vi "Target_4651.vi"() -> ()   [LabVIEW 2018]
uses:
  <vilib>/Platform/TimedLoop/XDataNode/timing_clust.ctl
  <vilib>/Platform/TimedLoop/XDataNode/nitl_modes.ctl
  <vilib>/Platform/TimedLoop/XDataNode/wakeup.ctl
  <vilib>/rvi/eio/common/nirviEmuTemplateMethod_errors.vi
  <vilib>/rvi/Emulation/niFpgaGetClockAttributes.vi
  <vilib>/rvi/Emulation/niFpgaSctlEmulationGetInTimedLoop.vi
  <vilib>/rvi/Emulation/niFpgaEmulationReportErrorSimple.vi
  <vilib>/rvi/Emulation/niFpgaProcessEmulError.vi
  <vilib>/rvi/Emulation/niFpgaCriticalErrorInLSC.vi
  <vilib>/rvi/Memory/Memory_Emulation/niFpgaMemoryFastEmulationDramWriteAndRequestData.vi
  <vilib>/rvi/Memory/Memory_Emulation/niFpgaMemoryEmulationDramWriteAndRequestData.vi
  <vilib>/rvi/DataTransferAndStorage/Container/Common/niFpgaContainerGetUniqueNameForEmu.vi
  <vilib>/rvi/Memory/Memory_Emulation/niFpgaMemoryEmulationDramWriteAndRequestDataApplyByteEnables.vi
  <vilib>/rvi/Memory/Memory_Emulation/nirvimemoryFastEmulation.vi
  <vilib>/rvi/Memory/Memory_Emulation/nirvimemoryEmulation.vi
  <vilib>/rvi/Emulation/niFpgaEmulationIsFPGAContextNoSignature.vi
  <vilib>/rvi/errors/nirviReportUnexpectedCaseInternalError (U32).vi
  <vilib>/rvi/interface/RandomDataEmulation/niFpgaRandomDataHandleErrors.vi
  <vilib>/eio/EIONode/EIONode.xnode
  <vilib>/Platform/TimedLoop/XDataNode/XDataNode.xnode
  <vilib>/rvi/DataTransferAndStorage/Container/XNode/niFpgaContainer.xnode
  <vilib>/rvi/interface/RandomDataEmulation/nirviRandomDataFpgaReadWriteTemplate.vi
  <vilib>/rvi/Memory/Memory_Emulation/niFpgaMemoryEmulationDramRetrieveData.vi
  <vilib>/Platform/TimedLoop/XDataNode/XDNodeRunTimeDep.lvlib
  <instrlib>/_niInstr/Basic Elements/v1/FPGA/niInstr Basic Elements v1 FPGA.lvlib
panel:
  in  "EOL":u64=281406257234029
  in  "SOL":u64=281406257234133
  in  "EOF":u64=281406257234105
  in  "SOF":u64=281406257233921
  in  "FR":u8=19
  in  "Кол-во":u16=370
  in  "Адрес":u16
  out "Записали адресов":u32
  in  "3924360":u32=3924360
  in  "48":u8=48
  in  "48":bool[](array[boolean])=[FALSE, FALSE, FALSE, FALSE, FALSE, FALSE, FALSE, FALSE, FALSE, FALSE, FALSE, FALSE, FALSE, FALSE, FALSE, FALSE, FALSE, FALSE, FALSE, FALSE, FALSE, FALSE, FALSE, FALSE, FALSE, FALSE, FALSE, FALSE, FALSE, FALSE, FALSE, FALSE, FALSE, FALSE, FALSE, FALSE, FALSE, FALSE, FALSE, FALSE, FALSE, FALSE, FALSE, FALSE, FALSE, FALSE, FALSE, FALSE]
  in  "Кадр в память":bool
  in  "Кадр на ПК":bool
  in  "Нач_адр":u32
  in  "Кон_адр":u32=32703
  out "Записали FIFO":bool
  in  "Автомат":bool
  in  "SYS_RST_N":bool
  in  "Стоп":bool
  out "SPI_OFF":bool
  in  "12":u8=12
  in  "W(T)/R(F)":bool
  in  "19":u8=19
  in  "SPI":bool
  in  "Upd_WR":bool
  in  "369":u16=369
  in  "Upd_RD":bool
  in  "372":u16=372
  in  "370":u16=370
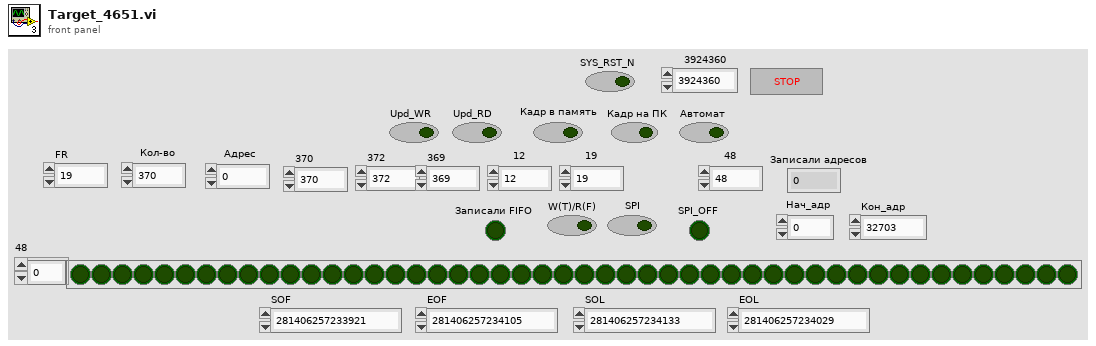
[diagram p1: front panel]
types:
  T1 = typedef "XDNodeRunTimeDep.lvlib/timing_clust.ctl" = cluster{"Expected End [f-1]":u64, "Actual End [f-1]":u64, "Finished Late? [f-1]":bool, "Expected End [i-1]":u64, "Actual End [i-1]":u64, "Finished Late? [i-1]":bool, "Expected Start [i]":u64, "Actual Start [i]":u64, "Expected Start [f]":u64, "Actual Start [f]":u64, "Source Name":string, "Structure Name":string, "Period":i64, "Deadline":i64, "Offset":i64, "Start":i64, "Priority":i32, "Timeout":i32, "Mode":T2, "Wakeup Reason":T3, "Error":errorcluster, "Source Type":string, "Secondary Source Type":string, "Global End Time":u64, "Global Start Time":u64, "Frame Duration":u64, "Iteration Duration":u64, "Assigned CPU":i32, "I/O Scan Engine Mode":u32}
  T2 = typedef "XDNodeRunTimeDep.lvlib/nitl_modes.ctl" = enum32{"No Change", "Process missed periods, maintain original phase", "Discard missed periods, maintain original phase", "Process missed periods, ignore original phase", "Discard missed periods, ignore original phase"}
  T3 = typedef "XDNodeRunTimeDep.lvlib/wakeup.ctl" = enum32{"Normal", "Aborted", "Asynchronous wakeup", "Timing source error", "Timed loop error", "Timeout"}
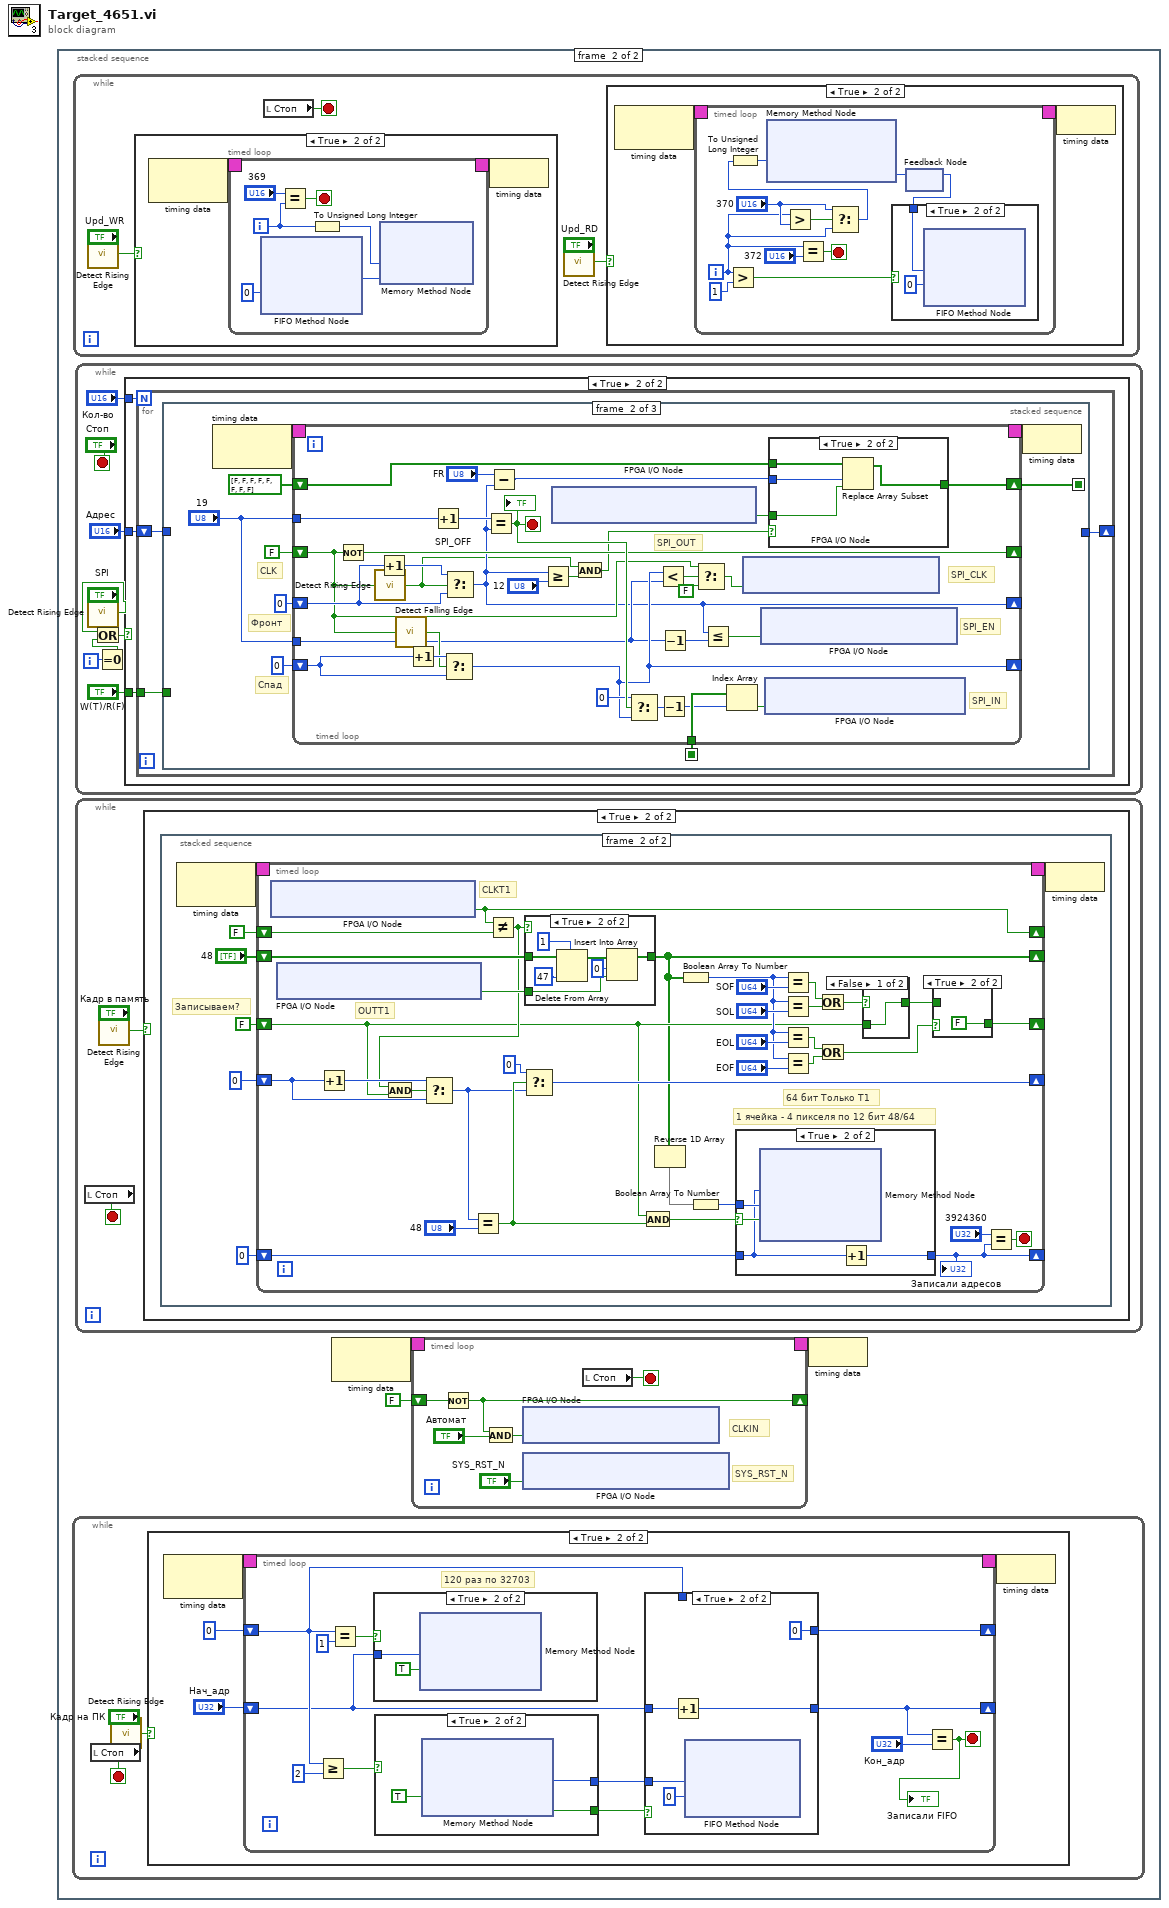
[diagram p0: block diagram]
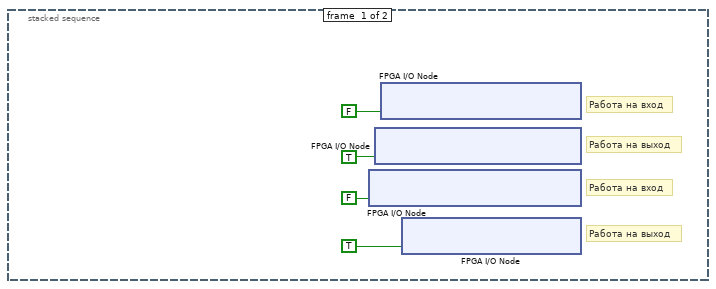
[diagram p2: hidden frame]
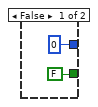
[diagram p4: hidden frame]
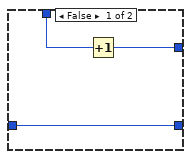
[diagram p6: hidden frame]
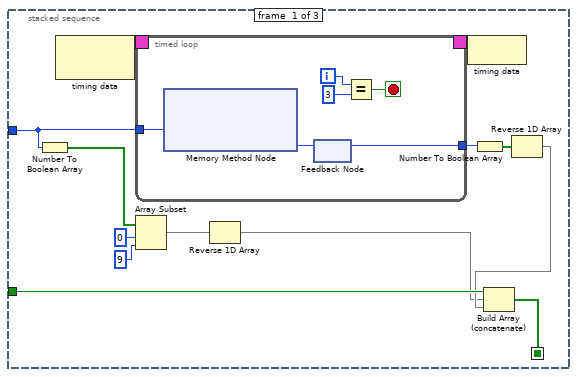
[diagram p11: hidden frame]
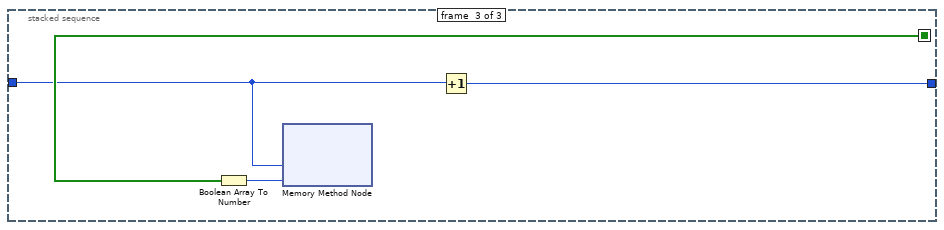
[diagram p13: hidden frame]
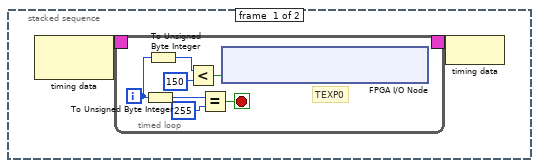
[diagram p15: hidden frame]
diagram:
  n1 = stacked-sequence {
    frame #0 {
      # "Работа на выход"
      # "Работа на вход"
      # "Работа на выход"
      # "Работа на вход"
      n2 = xnode "FPGA I/O Node"("IO Module\\DDCA_DIO16-23_WE"=FALSE ("IO Module\\DDCA_DIO16-23_WE")) -> ()  [unwired: 1 in, 1 out]
      n3 = xnode "FPGA I/O Node"("IO Module\\DDCA_DIO8-15_WE"=TRUE ("IO Module\\DDCA_DIO8-15_WE")) -> ()  [unwired: 1 in, 1 out]
      n4 = xnode "FPGA I/O Node"("IO Module\\DDCA_DIO0-7_WE"=FALSE ("IO Module\\DDCA_DIO0-7_WE")) -> ()  [unwired: 1 in, 1 out]
      n5 = xnode "FPGA I/O Node"("IO Module\\DDCA_PFI_WE"=TRUE ("IO Module\\DDCA_DIO16-23_WE")) -> ()  [unwired: 1 in, 1 out]
    }
    frame #1 {
      n6 = while {
        stop <- w10 stop-if-true
        n7 = local read "Стоп"() -> (w10:bool)
        n8 = call <instrlib>:"Detect Rising Edge.vi"("signal"="Кадр на ПК") -> ("edge detected"=w9:bool)  [unwired: 14 in]
        n9 = case shown="True" w9 {
          frame False {
          }
          frame True {
            n10 = node-c288() -> (w14:T1)  [unwired: 1 in]
            n11 = timed-loop {
              shift-right: [w25] -> _
              shift-left: "Нач_адр" -> [w16]
              timing: w14 -> [_]
              timing-out: [_] -> w13
              shift-right: [w18] -> _
              shift-left: u8 0 -> [w19]
              stop <- w26 stop-if-true
              # "120 раз по 32703"
              n12 = Greater Or Equal?(x=w19, y=u8 2 ("2")) -> (x >= y?=w20:bool)
              n13 = Equal?(x=w19, y=u8 1 ("1")) -> (x = y?=w23:bool)
              n14 = case shown="True" w23 {
                tunnel: w16 -> [_ w32]
                frame False {
                }
                frame True {
                  n15 = xnode ("Memory Method Node")("Address"=w32, "Input Valid"=TRUE) -> ()  [unwired: 1 in, 2 out]
                }
              }
              n16 = case shown="True" w20 {
                tunnel: [u8 0 ("Data") w31] -> w24
                tunnel: [FALSE ("Output Valid") w30] -> w15
                frame False {
                }
                frame True {
                  n17 = xnode ("Memory Method Node")("Ready for Output"=TRUE ("Ready For Output")) -> ("Data"=w31:u64, "Output Valid"=w30:bool)  [unwired: 1 in, 1 out]
                }
              }
              n18 = case shown="True" w15 {
                tunnel: [w34 w41] -> w25
                tunnel: w24 -> [_ w38]
                tunnel: w16 -> [w34 w40]
                tunnel: w19 -> [w36 _]
                tunnel: [w35 u8 0] -> w18
                frame False {
                  n19 = Increment(x=w36) -> (x+1=w35:u8)
                }
                frame True {
                  n20 = Increment(x=w40) -> (x+1=w41:u32)
                  n21 = xnode ("FIFO Method Node")("Element"=w38, "Timeout"=u8 0) -> ()  [unwired: 1 in, 2 out]
                }
              }
              n22 = Equal?(x=w25, y="Кон_адр") -> (x = y?=w26:bool)
              "Записали FIFO" <- w26
            }
            n23 = node-c288(w13) -> ()
          }
        }
      }
      n24 = while {
        stop <- w50 stop-if-true
        n25 = call <instrlib>:"Detect Rising Edge.vi"("signal"="Upd_WR") -> ("edge detected"=w48:bool)  [unwired: 14 in]
        n26 = case shown="True" w48 {
          frame False {
          }
          frame True {
            n27 = node-c288() -> (w71:T1)  [unwired: 1 in]
            n28 = timed-loop {
              timing: w71 -> [_]
              timing-out: [_] -> w70
              i -> [w75]
              stop <- w73 stop-if-true
              n29 = xnode ("FIFO Method Node")("Timeout"=u8 0) -> ("Element"=w72:u8)  [unwired: 1 in, 2 out]
              n30 = Equal?(x="369", y=w75) -> (x = y?=w73:bool)
              n31 = To Unsigned Long Integer(number=w75) -> (unsigned 32bit integer=w77:u32)
              n32 = xnode ("Memory Method Node")("Address"=w77, "Data"=w72) -> ()  [unwired: 1 in, 1 out]
            }
            n33 = node-c288(w70) -> ()
          }
        }
        n34 = local read "Стоп"() -> (w50:bool)
        n35 = call <instrlib>:"Detect Rising Edge.vi"("signal"="Upd_RD") -> ("edge detected"=w46:bool)  [unwired: 14 in]
        n36 = case shown="True" w46 {
          frame False {
          }
          frame True {
            n37 = node-c288() -> (w52:T1)  [unwired: 1 in]
            n38 = timed-loop {
              timing: w52 -> [_]
              timing-out: [_] -> w51
              i -> [w55]
              stop <- w58 stop-if-true
              n39 = Greater?(x=w55, y=u8 1) -> (0:w62:bool)
              n40 = Greater?(x=w55, y="370") -> (0:w57:bool)
              n41 = Equal?(x=w55, y="372") -> (x = y?=w58:bool)
              n42 = Select(t="370", s=w57, f=w55) -> (s? t:f=w54:i32)
              n43 = To Unsigned Long Integer(number=w54) -> (unsigned 32bit integer=w61:u32)
              n44 = xnode ("Memory Method Node")("Address"=w61) -> ("Data"=w60:u8)  [unwired: 2 in, 2 out]
              n45 = feedback #1() -> (w53:u8)  [unwired: 1 in]
              n46 = case shown="True" w62 {
                tunnel: w53 -> [_ w64]
                frame False {
                }
                frame True {
                  n47 = xnode ("FIFO Method Node")("Element"=w64, "Timeout"=u8 0) -> ()  [unwired: 1 in, 2 out]
                }
              }
              n48 = feedback-in #1(w60) -> ()
            }
            n49 = node-c288(w51) -> ()
          }
        }
      }
      n50 = while {
        i -> [w84]
        stop <- "Стоп" stop-if-true
        n51 = call <instrlib>:"Detect Rising Edge.vi"("signal"="SPI") -> ("edge detected"=w82:bool)  [unwired: 14 in]
        n52 = Equal To 0?(x=w84) -> (x = 0?=w83:bool)
        n53 = Or(x=w82, y=w83) -> (x .or. y?=w85:bool)
        n54 = case shown="True" w85 {
          tunnel: "W(T)/R(F)" -> [_ w93]
          tunnel: "Адрес" -> [_ w92]
          tunnel: "Кол-во" -> [_ w91]
          frame False {
          }
          frame True {
            n55 = for {
              N: w91 -> [_]
              tunnel: w93 -> [w96]
              shift-right: [w94] -> _
              shift-left: w92 -> [w95]
              n56 = stacked-sequence {
                seq-local: [w101 _ _] -> [_ w124 _]
                seq-local: [_ w122 _] -> [_ _ w172]
                tunnel: w96 -> [w103 _ _]
                tunnel: w95 -> [w100 _ w170]
                tunnel: [_ _ w173] -> w94
                frame #0 {
                  n57 = Number To Boolean Array(number=w100) -> (Boolean array=w99:bool[])
                  n58 = node-c288() -> (w109:T1)  [unwired: 1 in]
                  n59 = timed-loop {
                    timing: w109 -> [_]
                    timing-out: [_] -> w108
                    tunnel: w100 -> [w115]
                    tunnel: [w113] -> w107
                    i -> [w112]
                    stop <- w110 stop-if-true
                    n60 = xnode ("Memory Method Node")("Address"=w115) -> ("Data"=w114:u8)  [unwired: 1 in, 1 out]
                    n61 = feedback-in #2(w114) -> ()
                    n62 = feedback #2() -> (w113:u8)  [unwired: 1 in]
                    n63 = Equal?(x=w112, y=u8 3) -> (x = y?=w110:bool)
                  }
                  n64 = Array Subset(array=w99, index=0, length=9) -> (w98:bool[])
                  n65 = Reverse 1D Array(array=w98) -> (reversed array=w97:bool[])
                  n66 = node-c288(w108) -> ()
                  n67 = Number To Boolean Array(number=w107) -> (Boolean array=w106:bool[])
                  n68 = Reverse 1D Array(array=w106) -> (reversed array=w102:bool[])
                  n69 = Build Array (concatenate)(w103, w97, w102) -> (w101:bool[])
                }
                frame #1 {
                  # "Фронт"
                  # "Спад"
                  # "CLK"
                  n70 = node-c288() -> (w128:T1)  [unwired: 1 in]
                  n71 = timed-loop {
                    timing: w128 -> [_]
                    timing-out: [_] -> w127
                    shift-right: [w140] -> _
                    shift-left: FALSE -> [w139]
                    shift-right: [w145] -> _
                    shift-left: u8 0 -> [w148]
                    shift-right: [w133] -> _
                    shift-left: u8 0 -> [w159]
                    tunnel: "19" -> [w134]
                    tunnel: "19" -> [w150]
                    tunnel: w124 -> [w144]
                    shift-right: [w141] -> w122
                    shift-left: bool[] [FALSE, FALSE, FALSE, FALSE, FALSE, FALSE, FALSE, FALSE] -> [w142]
                    stop <- w147 stop-if-true
                    # "SPI_OUT"
                    # "SPI_IN"
                    # "SPI_CLK"
                    # "SPI_EN"
                    n72 = Not(x=w139) -> (.not. x?=w140:bool)
                    n73 = call <instrlib>:"Detect Rising Edge.vi"("signal"=w139) -> ("edge detected"=w131:bool)  [unwired: 14 in]
                    n74 = Increment(x=w159) -> (x+1=w160:u8)
                    n75 = call <instrlib>:"Detect Falling Edge.vi"("signal"=w139) -> ("edge detected"=w149:bool)  [unwired: 14 in]
                    n76 = Increment(x=w148) -> (x+1=w158:u8)
                    n77 = Increment(x=w150) -> (x+1=w151:u8)
                    n78 = Select(t=w158, s=w149, f=w148) -> (s? t:f=w145:u8)
                    n79 = Select(t=w160, s=w131, f=w159) -> (s? t:f=w133:u8)
                    n80 = Equal?(x=w151, y=w133) -> (x = y?=w147:bool)
                    "SPI_OFF" <- w147
                    n81 = Subtract(x="FR", y=w133) -> (x-y=w138:u8)
                    n82 = Greater Or Equal?(x=w133, y="12") -> (x >= y?=w132:bool)
                    n83 = xnode "FPGA I/O Node"() -> ("IO Module\\DDCA_DIO17_Read"=w153:bool)  [unwired: 1 in, 1 out]
                    n84 = And(x=w131, y=w132) -> (x .and. y?=w130:bool)
                    n85 = Select(t=u8 0, s=w147, f=w145) -> (s? t:f=w137:u8)
                    n86 = Less?(x=w145, y=w134) -> (x < y?=w156:bool)
                    n87 = Decrement(x=w137) -> (x-1=w136:u8)
                    n88 = Decrement(x=w134) -> (x-1=w135:u8)
                    n89 = Select(t=w139, s=w156, f=FALSE) -> (s? t:f=w154:bool)
                    n90 = Less Or Equal?(x=w133, y=w135) -> (x <= y?=w157:bool)
                    n91 = Index Array(array=w144, index=w136) -> (element=w143:bool)
                    n92 = xnode "FPGA I/O Node"("IO Module\\DDCA_PFI1_Write"=w154) -> ()  [unwired: 1 in, 1 out]
                    n93 = xnode "FPGA I/O Node"("IO Module\\DDCA_PFI3_Write"=w157) -> ()  [unwired: 1 in, 1 out]
                    n94 = xnode "FPGA I/O Node"("IO Module\\DDCA_DIO9_Write"=w143) -> ()  [unwired: 1 in, 1 out]
                    n95 = case shown="True" w130 {
                      tunnel: w153 -> [_ w164]
                      tunnel: w138 -> [_ w162]
                      tunnel: w142 -> [w161 w165]
                      tunnel: [w161 w163] -> w141
                      frame False {
                      }
                      frame True {
                        n96 = Replace Array Subset(array=w165, new element=w164, index=w162) -> (w163:bool[])
                      }
                    }
                  }
                  n97 = node-c288(w127) -> ()
                }
                frame #2 {
                  n98 = Boolean Array To Number(Boolean array=w172) -> (number=w171:u8)
                  n99 = xnode ("Memory Method Node")("Address"=w170, "Data"=w171) -> ()  [unwired: 2 in, 2 out]
                  n100 = Increment(x=w170) -> (x+1=w173:u16)
                }
              }
            }
          }
        }
      }
      n101 = while {
        stop <- w186 stop-if-true
        n102 = local read "Стоп"() -> (w186:bool)
        n103 = call <instrlib>:"Detect Rising Edge.vi"("signal"="Кадр в память") -> ("edge detected"=w185:bool)  [unwired: 14 in]
        n104 = case shown="True" w185 {
          frame False {
          }
          frame True {
            n105 = stacked-sequence {
              frame #0 {
                n106 = node-c288() -> (w188:T1)  [unwired: 1 in]
                n107 = timed-loop {
                  timing: w188 -> [_]
                  timing-out: [_] -> w187
                  i -> [w190]
                  stop <- w192 stop-if-true
                  # "TEXP0"
                  n108 = To Unsigned Byte Integer(number=w190) -> (unsigned 8bit integer=w189:u8)
                  n109 = To Unsigned Byte Integer(number=w190) -> (unsigned 8bit integer=w191:u8)
                  n110 = Less?(x=w191, y=u8 150) -> (x < y?=w193:bool)
                  n111 = Equal?(x=w189, y=u8 255) -> (x = y?=w192:bool)
                  n112 = xnode "FPGA I/O Node"("IO Module\\DDCA_DIO13_Write"=w193) -> ()  [unwired: 1 in, 1 out]
                }
                n113 = node-c288(w187) -> ()
              }
              frame #1 {
                # "Записываем?"
                n114 = node-c288() -> (w206:T1)  [unwired: 1 in]
                n115 = timed-loop {
                  shift-right: [w240] -> _
                  shift-left: FALSE -> [w241]
                  shift-right: [w208] -> _
                  shift-left: "48" -> [w237]
                  timing: w206 -> [_]
                  timing-out: [_] -> w205
                  shift-right: [w238] -> _
                  shift-left: u32 0 -> [w239]
                  shift-right: [w226] -> _
                  shift-left: FALSE -> [w211]
                  shift-right: [w214] -> _
                  shift-left: u8 0 -> [w217]
                  stop <- w220 stop-if-true
                  # "1 ячейка - 4 пикселя по 12 бит 48/64"
                  # "64 бит Только Т1"
                  # "CLKT1"
                  # "OUTT1"
                  n116 = xnode "FPGA I/O Node"() -> ("IO Module\\DDCA_DIO23_Read"=w240:bool)  [unwired: 1 in, 1 out]
                  n117 = xnode "FPGA I/O Node"() -> ("IO Module\\DDCA_DIO21_Read"=w236:bool)  [unwired: 1 in, 1 out]
                  n118 = Increment(x=w217) -> (x+1=w218:u8)
                  n119 = Not Equal?(x=w240, y=w241) -> (x != y?=w212:bool)
                  n120 = And(x=w212, y=w211) -> (x .and. y?=w210:bool)
                  n121 = Select(t=w218, s=w210, f=w217) -> (s? t:f=w213:u8)
                  n122 = Equal?(x=w213, y="48") -> (x = y?=w216:bool)
                  n123 = Select(t=u8 0, s=w216, f=w213) -> (s? t:f=w214:u8)
                  n124 = case shown="True" w212 {
                    tunnel: w237 -> [w251 w254]
                    tunnel: w236 -> [_ w257]
                    tunnel: [w251 w256] -> w208
                    frame False {
                    }
                    frame True {
                      n125 = Delete From Array(array=w254, length=1, index=47) -> (array with subset deleted=w255:bool[])  [unwired: 1 out]
                      n126 = Insert Into Array(array=w255, index=u8 0, new element=w257) -> (w256:bool[])
                    }
                  }
                  n127 = And(x=w211, y=w216) -> (x .and. y?=w219:bool)
                  n128 = Reverse 1D Array(array=w208) -> (reversed array=w207:bool[])
                  n129 = Boolean Array To Number(Boolean array=w208) -> (number=w222:u64)
                  n130 = Boolean Array To Number(Boolean array=w207) -> (number=w209:u64)
                  n131 = case shown="True" w219 {
                    selector: w219 -> [_ w244]
                    tunnel: [w242 w246] -> w238
                    tunnel: w209 -> [_ w245]
                    tunnel: w239 -> [w242 w243]
                    frame False {
                    }
                    frame True {
                      n132 = xnode ("Memory Method Node")("Address"=w243, "Data"=w245, "Input Valid"=w244) -> ()  [unwired: 1 in, 2 out]
                      n133 = Increment(x=w243) -> (x+1=w246:u32)
                    }
                  }
                  "Записали адресов" <- w238
                  n134 = Equal?(x=w222, y="SOF") -> (x = y?=w233:bool)
                  n135 = Equal?(x=w222, y="SOL") -> (x = y?=w232:bool)
                  n136 = Equal?(x=w222, y="EOL") -> (x = y?=w230:bool)
                  n137 = Equal?(x=w222, y="EOF") -> (x = y?=w229:bool)
                  n138 = Or(x=w233, y=w232) -> (x .or. y?=w231:bool)
                  n139 = Or(x=w230, y=w229) -> (x .or. y?=w228:bool)
                  n140 = case shown="False" w231 {
                    selector: w231 -> [_ w250]
                    tunnel: [w249 w250] -> w227
                    tunnel: w211 -> [w249 _]
                    frame False {
                    }
                    frame True {
                    }
                  }
                  n141 = case shown="True" w228 {
                    tunnel: [w247 FALSE] -> w226
                    tunnel: w227 -> [w247 _]
                    frame False {
                    }
                    frame True {
                    }
                  }
                  n142 = Equal?(x="3924360", y=w238) -> (x = y?=w220:bool)
                }
                n143 = node-c288(w205) -> ()
              }
            }
          }
        }
      }
      n144 = node-c288() -> (w7:T1)  [unwired: 1 in]
      n145 = timed-loop {
        timing: w7 -> [_]
        timing-out: [_] -> w6
        shift-right: [w174] -> _
        shift-left: FALSE -> [w178]
        stop <- w179 stop-if-true
        # "SYS_RST_N"
        # "CLKIN"
        n146 = Not(x=w178) -> (.not. x?=w174:bool)
        n147 = And(x=w174, y="Автомат") -> (x .and. y?=w175:bool)
        n148 = xnode "FPGA I/O Node"("IO Module\\DDCA_PFI2_Write"=w175) -> ()  [unwired: 1 in, 1 out]
        n149 = xnode "FPGA I/O Node"("IO Module\\DDCA_DIO11_Write"="SYS_RST_N") -> ()  [unwired: 1 in, 1 out]
        n150 = local read "Стоп"() -> (w179:bool)
      }
      n151 = node-c288(w6) -> ()
    }
  }
